vi "setDescription.vi"(8 "error in (no error)":errorcluster, 10 "Description in":string, 11 "IComponent in":refnum<class "IComponent.lvclass">) -> (0 "error out":errorcluster, 3 "IComponent out":refnum<class "IComponent.lvclass">)   [LabVIEW 2022 SP3, in "openDAQ.lvlib" / "IBaseObject.lvlib" / "IPropertyObject.lvlib" / "IComponent.lvlib" / "IComponent.lvclass"]
uses:
  <instrlib>/openDAQ/Public/Classes/IComponent/IComponent.lvclass
  <instrlib>/openDAQ/Public/Classes/IComponent/IComponent.lvclass/IComponent.ctl
  <instrlib>/openDAQ/Public/Classes/daqCoreTypes/IString/IString.lvclass
  <instrlib>/openDAQ/Binaries/Windows/x86/copendaq32.dll
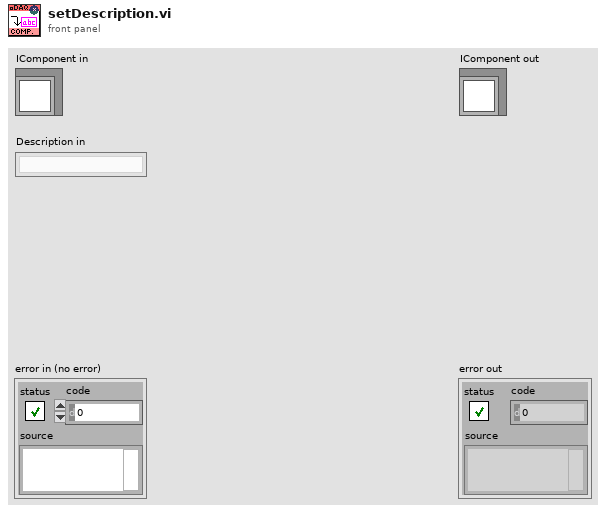
[diagram p1: front panel]
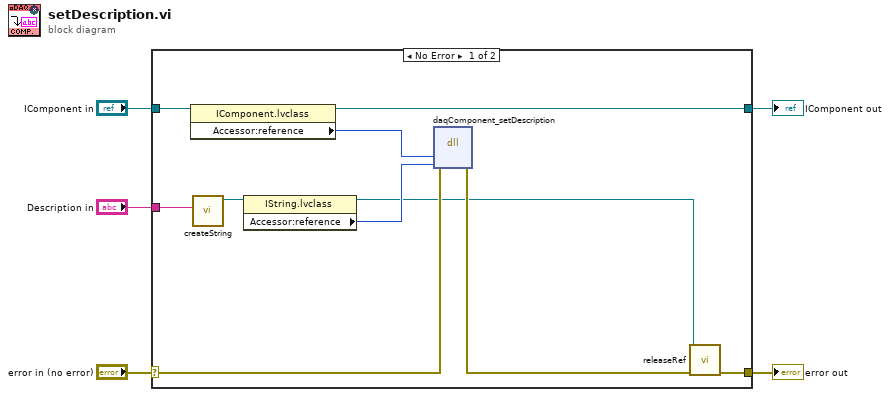
[diagram p0: block diagram]
diagram:
  n1 = case shown="No Error" "error in (no error)" {
    selector: "error in (no error)" -> [w13 w17]
    tunnel: [w7 w17] -> w4
    tunnel: [w14 w16] -> w2
    tunnel: "IComponent in" -> [w15 w16]
    tunnel: "Description in" -> [w11 _]
    frame No Error {
      n2 = property class="IComponent.lvclass"(reference=w15) -> (reference out=w14:refnum<class "IComponent.lvclass">, "Accessor:reference"=w10:i64)  [unwired: 1 in, 1 out]
      n3 = call <instrlib>:"createString.vi"("String"=w11) -> ("IString out"=w12:refnum<class "IString.lvclass">)  [unwired: 9 in, 1 out]
      n4 = property class="IString.lvclass"(reference=w12) -> (reference out=w6:refnum<class "IString.lvclass">, "Accessor:reference"=w9:i64)  [unwired: 1 in, 1 out]
      n5 = dll-call lib="C:/Program Files (x86)/National Instruments/LabVIEW 2022/instr.lib/openDAQ/Binaries/Windows/x86/copendaq*.*" fn="daqComponent_setDescription"(error in=w13, "component"=w10, "description"=w9) -> (error out=w8:errorcluster)  [unwired: 5 in, 1 out]
      n6 = call-dynamic "releaseRef.vi"("error in (no error)"=w8, "IBaseObject in"=w6) -> ("error out"=w7:errorcluster)  [unwired: 9 in]
    }
    frame Error {
    }
  }
  "error out" <- w4
  "IComponent out" <- w2
